vi "read_from_text_file.vi"(7 "delimiter (\\t)":string="\t", 8 "error in (no error)":errorcluster, 10 "file (use dialog)":path, 11 "PointCollection in":refnum<class "PointCollection.lvclass">) -> (0 "error out":errorcluster, 3 "PointCollection out":refnum<class "PointCollection.lvclass">)   [LabVIEW 2010, in "PointCollection.lvclass"]
uses:
  PointCollection.lvclass
  mode_enum.ctl
  <vilib>/Utility/file.llb/Read From Spreadsheet File (DBL).vi
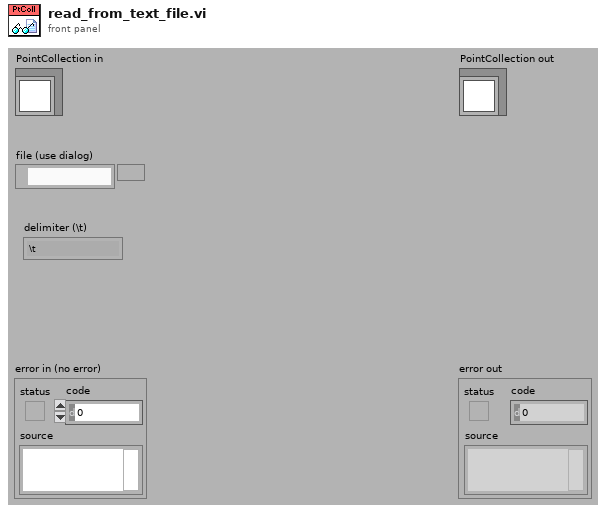
[diagram p1: front panel]
types:
  T1 = typedef "PointCollection.lvclass/mode_enum.ctl" = enum16{"points first", "dimensions first"}
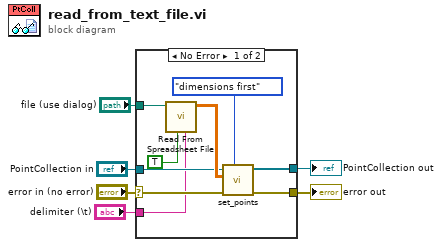
[diagram p0: block diagram]
diagram:
  n1 = case shown="No Error" "error in (no error)" {
    selector: "error in (no error)" -> [w14 w17]
    tunnel: [w13 w17] -> w5
    tunnel: [w11 w16] -> w3
    tunnel: "PointCollection in" -> [w12 w16]
    tunnel: "file (use dialog)" -> [w10 _]
    tunnel: "delimiter (\\t)" -> [w9 _]
    frame No Error {
      n2 = call-poly <vilib>:"Read From Spreadsheet File.vi"("delimiter (\\t)"=w9, "transpose (no:F)"=TRUE, "file path (dialog if empty)"=w10) -> ("all rows"=w15:dbl[][])  [unwired: 4 in, 4 out]
      n3 = call "set_points.vi"("mode"=mode_enum."dimensions first", "error in (no error)"=w14, "points (dimensions/points)"=w15, "PointCollection in"=w12) -> ("error out"=w13:errorcluster, "PointCollection out"=w11:refnum<class "PointCollection.lvclass">)  [unwired: 6 in]
    }
    frame Error {
    }
  }
  "error out" <- w5
  "PointCollection out" <- w3
